vi "ExSubCol2Nframe.vi"(1 "error in (no error)":errorcluster, 2 "Number of Images":u32=1 min=1 step=1, 3 "Handle Cluster Camera 2":T1, 4 "Handle Cluster Camera 1":T1) -> (0 "error out":errorcluster)   [LabVIEW 2010]
panel:
  # "ExSubCol2Nframe.vi : this sub vi collects n frames from \ntwo cameras."
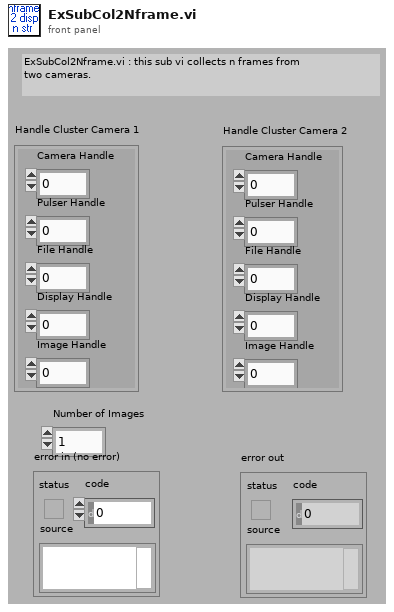
[diagram p1: front panel]
types:
  T1 = cluster{"Camera Handle":u32, "Pulser Handle":u32, "File Handle":u32, "Display Handle":u32, "Image Handle":u32}
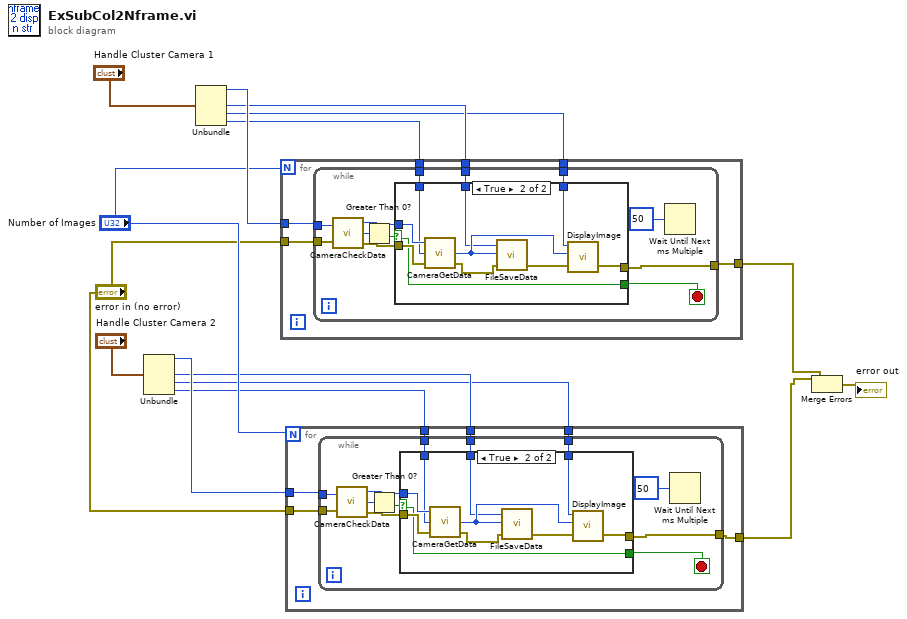
[diagram p0: block diagram]
diagram:
  n1 = Unbundle("Handle Cluster Camera 2") -> ("Camera Handle"=w10:u32, "File Handle"=w9:u32, "Display Handle"=w8:u32, "Image Handle"=w7:u32)  [unwired: 1 out]
  n2 = Unbundle("Handle Cluster Camera 1") -> ("Camera Handle"=w15:u32, "File Handle"=w14:u32, "Display Handle"=w13:u32, "Image Handle"=w12:u32)  [unwired: 1 out]
  n3 = for {
    N: "Number of Images" -> [_]
    tunnel: w15 -> [w21]
    tunnel: w14 -> [w20]
    tunnel: w13 -> [w19]
    tunnel: w12 -> [w18]
    tunnel: "error in (no error)" -> [w17]
    tunnel: [w16] -> w3
    n4 = while {
      tunnel: w21 -> [w32]
      tunnel: [w27] -> w16
      tunnel: w20 -> [w26]
      tunnel: w19 -> [w25]
      tunnel: w18 -> [w24]
      tunnel: w17 -> [w22]
      stop <- w28 stop-if-true
      n5 = call <userlib>:"CameraCheckData.vi"("Camera Handle"=w32, "error in"=w22) -> ("Camera Handle"=w30:u32, "Number Of Frames Available"=w33:i32, "error out"=w29:errorcluster)
      n6 = Greater Than 0?(x=w33) -> (x > 0?=w31:bool)
      n7 = case shown="True" w31 {
        selector: w31 -> [w34 w43]
        tunnel: w30 -> [_ w45]
        tunnel: w29 -> [w35 w44]
        tunnel: [w34 w43] -> w28
        tunnel: [w35 w40] -> w27
        tunnel: w26 -> [_ w38]
        tunnel: w25 -> [_ w37]
        tunnel: w24 -> [_ w36]
        frame False {
        }
        frame True {
          n8 = call <userlib>:"CameraGetData.vi"("error in"=w44, "Data Handle"=w36, "Camera Handle"=w45) -> ("error out"=w42:errorcluster, "Data Handle"=w39:u32)  [unwired: 1 out]
          n9 = call <userlib>:"FileSaveData.vi"("error in"=w42, "Image Handle"=w39, "File Handle"=w38) -> ("error out"=w41:errorcluster)  [unwired: 1 out]
          n10 = call <userlib>:"DisplayImage.vi"("error in"=w41, "Image Handle"=w39, "Display Handle"=w37) -> ("error out"=w40:errorcluster)  [unwired: 1 in, 1 out]
        }
      }
      n11 = Wait Until Next ms Multiple(millisecond multiple=u32 50) -> ()  [unwired: 1 out]
    }
  }
  n12 = for {
    N: "Number of Images" -> [_]
    tunnel: w10 -> [w51]
    tunnel: w9 -> [w50]
    tunnel: w8 -> [w49]
    tunnel: w7 -> [w48]
    tunnel: "error in (no error)" -> [w47]
    tunnel: [w46] -> w2
    n13 = while {
      tunnel: w51 -> [w62]
      tunnel: [w57] -> w46
      tunnel: w50 -> [w56]
      tunnel: w49 -> [w55]
      tunnel: w48 -> [w54]
      tunnel: w47 -> [w52]
      stop <- w58 stop-if-true
      n14 = call <userlib>:"CameraCheckData.vi"("Camera Handle"=w62, "error in"=w52) -> ("Camera Handle"=w60:u32, "Number Of Frames Available"=w63:i32, "error out"=w59:errorcluster)
      n15 = Greater Than 0?(x=w63) -> (x > 0?=w61:bool)
      n16 = case shown="True" w61 {
        selector: w61 -> [w64 w73]
        tunnel: w60 -> [_ w75]
        tunnel: w59 -> [w65 w74]
        tunnel: [w64 w73] -> w58
        tunnel: [w65 w70] -> w57
        tunnel: w56 -> [_ w68]
        tunnel: w55 -> [_ w67]
        tunnel: w54 -> [_ w66]
        frame False {
        }
        frame True {
          n17 = call <userlib>:"CameraGetData.vi"("error in"=w74, "Data Handle"=w66, "Camera Handle"=w75) -> ("error out"=w72:errorcluster, "Data Handle"=w69:u32)  [unwired: 1 out]
          n18 = call <userlib>:"FileSaveData.vi"("error in"=w72, "Image Handle"=w69, "File Handle"=w68) -> ("error out"=w71:errorcluster)  [unwired: 1 out]
          n19 = call <userlib>:"DisplayImage.vi"("error in"=w71, "Image Handle"=w69, "Display Handle"=w67) -> ("error out"=w70:errorcluster)  [unwired: 1 in, 1 out]
        }
      }
      n20 = Wait Until Next ms Multiple(millisecond multiple=u32 50) -> ()  [unwired: 1 out]
    }
  }
  n21 = Merge Errors(w3, w2) -> (→"error out":errorcluster)
